vi "angle Converter.vi"(7 "select":enum16{"-180~180", "0~360"}(ring), 9 "input angle":dbl) -> (1 "angle out":dbl)   [LabVIEW 2019, in "angle Converter.lvclass"]
uses:
  angle Converter.lvclass
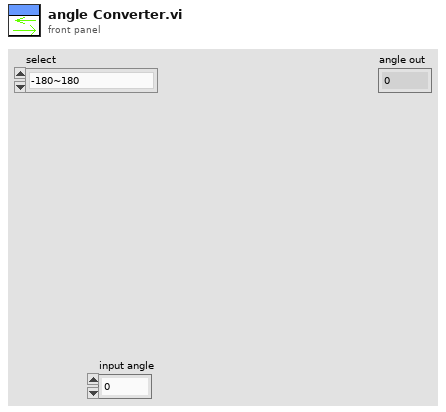
[diagram p1: front panel]
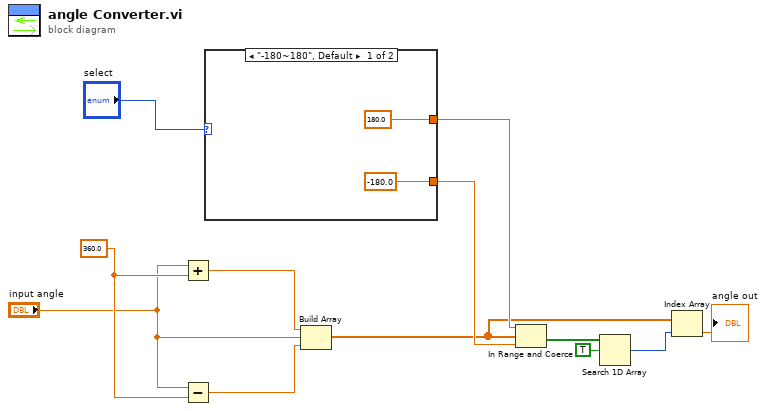
[diagram p0: block diagram]
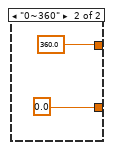
[diagram p2: hidden frame]
diagram:
  w12 = 360.0
  n1 = Add(x="input angle", y=w12) -> (x+y=w10:dbl)
  n2 = Subtract(x="input angle", y=w12) -> (x-y=w9:dbl)
  n3 = case shown="\"-180~180\", Default" "select" {
    tunnel: [180.0 360.0] -> w7
    tunnel: [-180.0 0.0] -> w6
    frame "-180~180", Default {
    }
    frame "0~360" {
    }
  }
  n4 = Build Array(w10, "input angle", w9) -> (w2:dbl[])
  n5 = In Range and Coerce(upper limit=w7, x=w2, lower limit=w6) -> (In Range?=w5:bool[])  [unwired: 1 out]
  n6 = Search 1D Array(1D array=w5, element=TRUE) -> (index of element=w4:i32)  [unwired: 1 in]
  n7 = Index Array(array=w2, index=w4) -> (element=→"angle out":dbl)
